vi "stopSnapping.vi"(8 "error in (no error)":errorcluster, 11 "CameraManager in":refnum<class "CameraManager.lvclass">) -> (0 "error out":errorcluster, 3 "CameraManager out":refnum<class "CameraManager.lvclass">)   [LabVIEW 2011, in "iManagement.lvlib" / "CameraManager.lvclass"]
uses:
  CameraManager.lvclass
  CameraManager.lvclass/CameraManager.ctl
  Hal/Channels/Camera/CameraController.lvclass
  Hal/Channels/Camera/CameraEventsManager/CameraEventsManger.lvclass
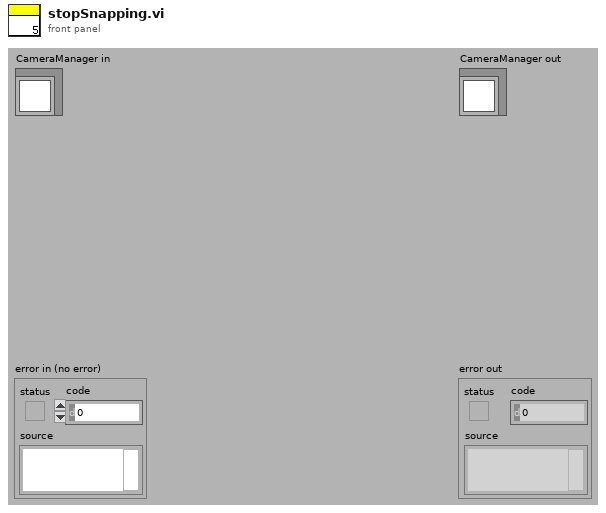
[diagram p1: front panel]
types:
  T1 = cluster{"frontEndEvents":cluster{"snapShotEvent":refnum<user-event>, "stopShooting":refnum<user-event>, "userSnapShot":refnum<user-event>}, "backEndEvents":cluster{"picture":refnum<user-event>}}
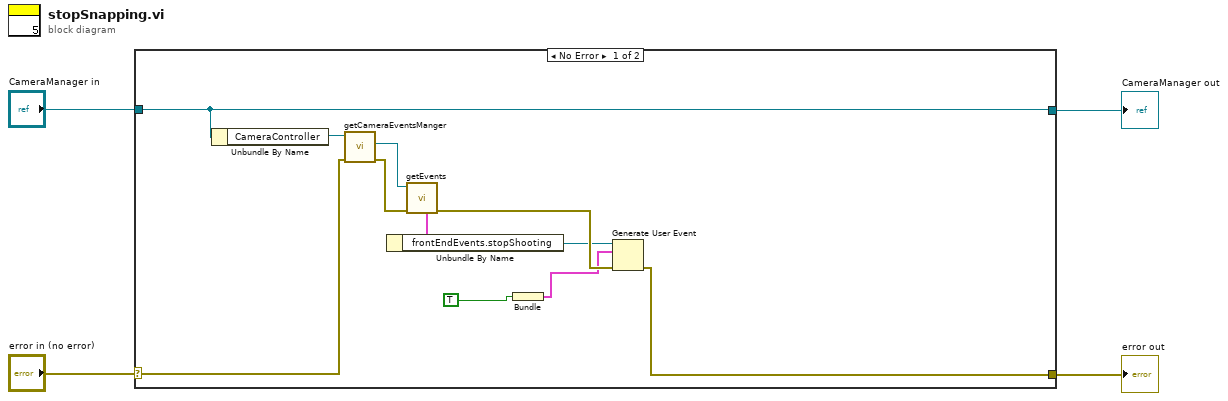
[diagram p0: block diagram]
diagram:
  n1 = case shown="No Error" "error in (no error)" {
    selector: "error in (no error)" -> [w9 w17]
    tunnel: [w7 w17] -> w3
    tunnel: [w10 w16] -> w1
    tunnel: "CameraManager in" -> [w10 w16]
    frame No Error {
      n2 = Unbundle By Name(w10) -> ("CameraController"=w13:refnum<class "CameraController.lvclass">)
      n3 = call-dynamic "getCameraEventsManger.vi"("error in (no error)"=w9, "CameraController.lvclass in"=w13) -> ("error out"=w14:errorcluster, "Hardware:Channels.lvlib:CameraEventsManger.lvclass"=w15:refnum<class "CameraEventsManger.lvclass">)  [unwired: 7 in, 1 out]
      n4 = call-dynamic "getEvents.vi"("error in (no error)"=w14, "CameraEventsManger in"=w15) -> ("error out"=w11:errorcluster, "snapperEvents"=w12:T1)  [unwired: 5 in, 3 out]
      n5 = Unbundle By Name(w12) -> ("frontEndEvents.stopShooting"=w8:refnum<user-event>)
      n6 = Bundle(TRUE) -> (w5:cluster{bool})  [unwired: 1 in]
      n7 = Generate User Event(user event=w8, event data cluster=w5, error in=w11) -> (error out=w7:errorcluster)  [unwired: 1 out]
    }
    frame Error {
    }
  }
  "error out" <- w3
  "CameraManager out" <- w1
